vi "test Disabled Device Can Be Deployed.vi"(8 "error in (no error)":errorcluster, 11 "Deployment in":refnum<class "Deployment.lvclass">) -> (0 "error out":errorcluster, 3 "Deployment out":refnum<class "Deployment.lvclass">)   [LabVIEW 2020, in "Deployment.lvclass"]
uses:
  Deployment.lvclass
  Deployment.lvclass/Deployment.ctl
  <vilib>/addons/_JKI Toolkits/VI Tester/TestCase.llb/TestCase.lvclass
  niveristand-custom-device-testing-tools/VeriStandTestUtilities/VeriStandTestUtilities.lvlib
  Scripting/Ballard/Ballard ARINC 429 Scripting.lvlib
  C:/Program Files (x86)/National Instruments/LabVIEW 2020/vi.lib/addons/_JKI Toolkits/VI Tester/TestCase.llb/TestCase.lvclass
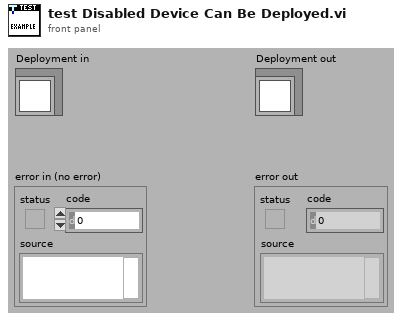
[diagram p1: front panel]
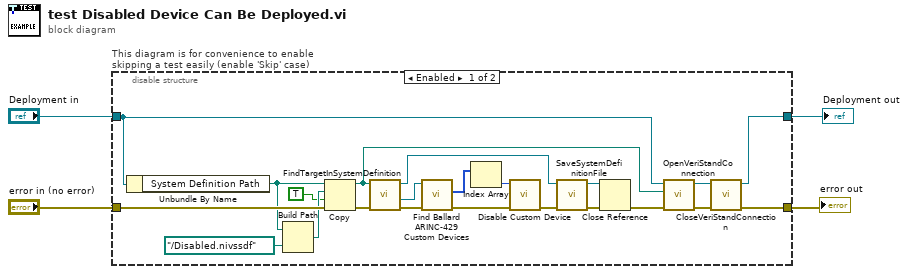
[diagram p0: block diagram]
diagram:
  n1 = disable-structure "This diagram is for convenience to enable skipping a test easily (enable 'Skip' case)" shown="Enabled" {
    disable-tunnel: "Deployment in" -> [w22 w30]
    disable-tunnel: [w23 w28] -> w1
    disable-tunnel: [w24 w29] -> w3
    disable-tunnel: "error in (no error)" -> [w21 w27]
    frame Enabled {
      n2 = Unbundle By Name(w22) -> ("System Definition Path"=w18:path)
      n3 = Build Path(base path=w18, name or relative path=path "../Disabled.nivssdf") -> (appended path=w19:path)
      n4 = Copy(8:w21, 9:TRUE ("overwrite (F)"), 10:w19, 11:w18) -> (0:w20:errorcluster, 3:w6:path)  [unwired: 1 in, 1 out]
      n5 = call "FindTargetInSystemDefinition.vi"("error in"=w20, "system definition path"=w6) -> ("error out"=w16:errorcluster, "Target"=w15:refnum<k24>, "System Definition"=w10:refnum<k24>)  [unwired: 6 in, 1 out]
      n6 = call "Find Ballard ARINC-429 Custom Devices.vi"("error in"=w16, "target in"=w15) -> ("error out"=w12:errorcluster, "Ballard ARINC 429 custom devices"=w14:u64[])  [unwired: 7 in, 1 out]
      n7 = Index Array(array=w14) -> (element=w13:u64)  [unwired: 1 in]
      n8 = call "Disable Custom Device.vi"("error in (no error)"=w12, "Ballard ARINC 429 ref"=w13) -> ("error out"=w11:errorcluster)  [unwired: 8 in, 1 out]
      n9 = call "SaveSystemDefinitionFile.vi"("error in (no error)"=w11, "System Definition Reference in"=w10) -> ("error out"=w9:errorcluster, "System Definition Reference out"=w8:refnum<k24>)  [unwired: 8 in]
      n10 = Close Reference(reference=w8, error in (no error)=w9) -> (error out=w7:errorcluster)
      n11 = call-dynamic "OpenVeriStandConnection.vi"("error in (no error)"=w7, "System Definition File"=w6, "VeriStand Test Case in"=w22) -> ("error out"=w26:errorcluster, "VeriStand Test Case out"=w25:refnum<class "Deployment.lvclass">)  [unwired: 6 in, 1 out]
      n12 = call-dynamic "CloseVeriStandConnection.vi"("error in (no error)"=w26, "VeriStand Test Case in"=w25) -> ("error out"=w24:errorcluster, "VeriStand Test Case out"=w23:refnum<class "Deployment.lvclass">)  [unwired: 8 in]
    }
    frame Disabled {
      # "skip test result while test is under development"
      n13 = call <vilib>:"skip.vi"("error in (no error)"=w27, "TestCase in"=w30) -> ("error out"=w29:errorcluster, "TestCase out"=w28:refnum<class "Deployment.lvclass">)  [unwired: 8 in]
    }
  }
  "error out" <- w3
  "Deployment out" <- w1
